vi "Read hardware channels.vi"(8 "error in (no error)":errorcluster, 11 "Rx Execution Unit in":refnum<class "Rx Execution Unit.lvclass">) -> (0 "error out":errorcluster, 2 "hardware channels":T1[](array[typedef]) {"channel settings"."Cluster"."DefaultCronoMode" items=["FDX_RX_DEFAULT_ENA_CNT", "FDX_RX_DEFAULT_MON_ENA_ALL", "FDX_RX_DEFAULT_MON_ENA_GOOD"]}, 3 "Rx Execution Unit out":refnum<class "Rx Execution Unit.lvclass">)   [LabVIEW 2020, in "afdx_custom_device Engine.lvlib" / "Implementation.lvlib" / "Rx Execution Unit.lvclass"]
uses:
  Rx Execution Unit.lvclass
  AIM LabVIEW src/src/_controls/session_monitor_config.ctl
  AIM LabVIEW src/src/AIM664LV.lvlib
  channel_settings_rx.ctl
  hardware_channels_rx.ctl
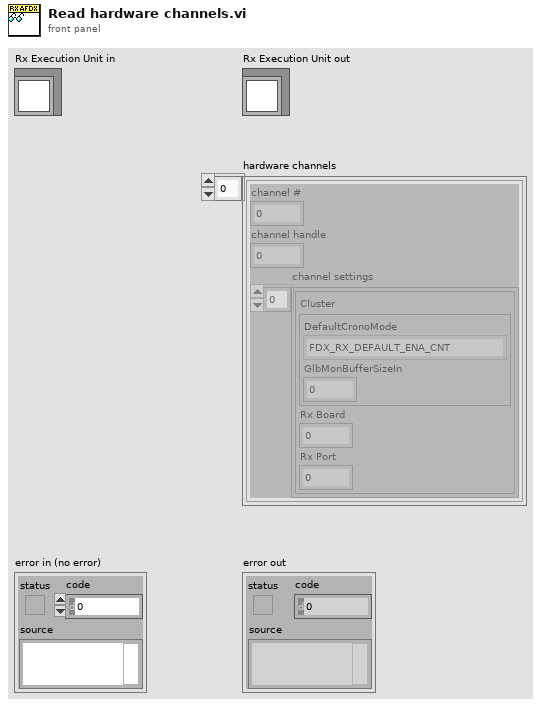
[diagram p1: front panel]
types:
  T1 = typedef "hardware_channels_rx.ctl" = cluster{"channel #":u16, "channel handle":u64, "channel settings":T2[]}
  T2 = typedef "channel_settings_rx.ctl" = cluster{"Cluster":T3, "Rx Board":dbl, "Rx Port":dbl}
  T3 = typedef "AIM664LV.lvlib/session_monitor_config.ctl" = cluster{"DefaultCronoMode":u32, "GlbMonBufferSizeIn":u32}
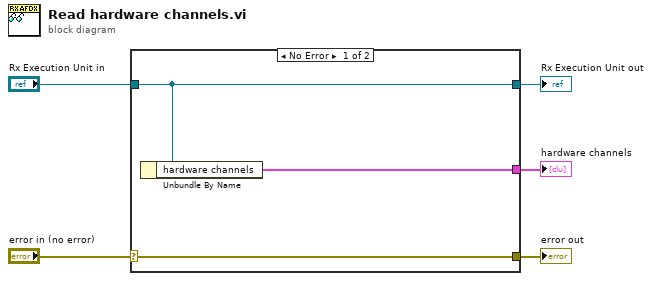
[diagram p0: block diagram]
diagram:
  n1 = case shown="No Error" "error in (no error)" {
    selector: "error in (no error)" -> [w8 w9]
    tunnel: [w8 w9] -> w4
    tunnel: [w7 w10] -> w2
    tunnel: "Rx Execution Unit in" -> [w7 w10]
    tunnel: [w6 _] -> w1
    frame No Error {
      n2 = Unbundle By Name(w7) -> ("hardware channels"=w6:T1[])
    }
    frame Error {
    }
  }
  "error out" <- w4
  "Rx Execution Unit out" <- w2
  "hardware channels" <- w1
